vi "Max_&_Min_Array_1D.vi"(11 "Max & Min Array 1D":i8[](array[numeric])=[1, -1, 2, 100, 10]) -> (0 "Index Min.":i32, 1 "Min. Value":i8, 2 "Index Max.":i32, 3 "Max. Value":i8)   [LabVIEW 2018]
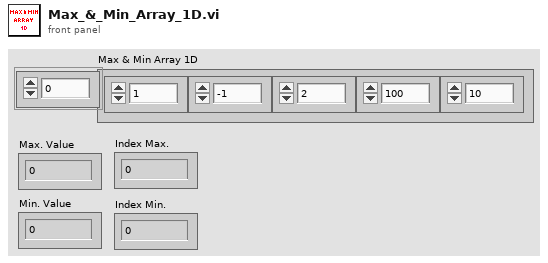
[diagram p1: front panel]
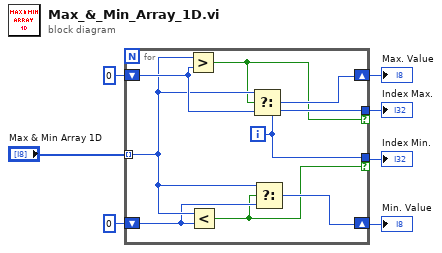
[diagram p0: block diagram]
diagram:
  n1 = for {
    tunnel: "Max & Min Array 1D" -> [w13] mode=indexing
    shift-right: [w14] -> w1
    shift-left: i8 0 -> [w15]
    shift-right: [w9] -> w2
    shift-left: i8 0 -> [w12]
    tunnel: [w11] -> w5 if=w10
    tunnel: [w11] -> w4 if=w8
    i -> [w11]
    n2 = Greater?(x=w13, y=w15) -> (0:w10:bool)
    n3 = Less?(x=w13, y=w12) -> (x < y?=w8:bool)
    n4 = Select(t=w13, s=w10, f=w15) -> (s? t:f=w14:i8)
    n5 = Select(t=w13, s=w8, f=w12) -> (s? t:f=w9:i8)
  }
  "Max. Value" <- w1
  "Index Max." <- w5
  "Index Min." <- w4
  "Min. Value" <- w2
